vi "LoadProfile.vi"(0 "path":string, 5 "error in":T1) -> (14 "path out":string, 19 "error out":T1)   [LabVIEW 2016]
doc: "Loads the settings of an existing profile which is stored at \"path\" into the controller."
uses:
  Controls/Error_Out.ctl
  Files_ASC500/DLL/ASC500_RemoteControlV27.dll
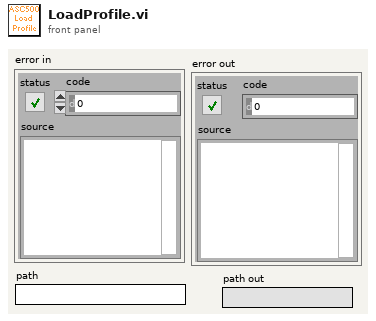
[diagram p1: front panel]
types:
  T1 = typedef "Error_Out.ctl" = errorcluster
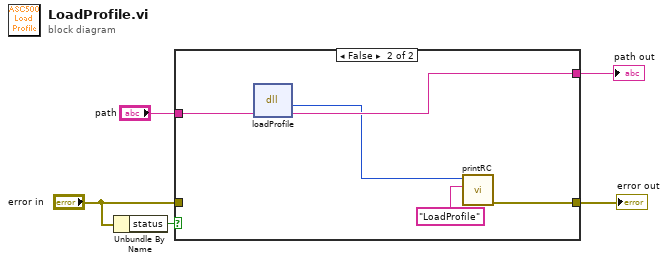
[diagram p0: block diagram]
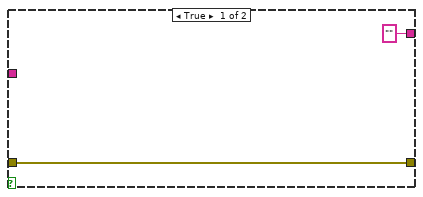
[diagram p2: hidden frame]
diagram:
  n1 = Unbundle By Name("error in") -> ("status"=w4:bool)
  n2 = case shown="False" w4 {
    tunnel: [w6 w9] -> w5
    tunnel: "path" -> [_ w12]
    tunnel: ["" ("Path") w11] -> w2
    tunnel: "error in" -> [w6 _]
    frame True {
    }
    frame False {
      n3 = dll-call lib="G:/SCMOperations/Share/ELE/Produkt Information/ASC500/04 Remote Control/02 development versions/2018Nov06/Files_ASC500/DLL/ASC500_RemoteControlV27.dll" fn="loadProfile"("Path"=w12) -> ("Rückgabetyp"=w10:i32, "Path"=w11:string)  [unwired: 3 in, 2 out]
      n4 = call "printRC.vi"("additional information"="LoadProfile", "RC"=w10) -> ("error out"=w9:T1)  [unwired: 9 in]
    }
  }
  "error out" <- w5
  "path out" <- w2
